vi "Send DB Data.vi"(0 "error in":errorcluster) -> ()   [LabVIEW 2012]
uses:
  Systems/Cannon/Cannon Global Data.vi
  Systems/Conveyer Belt/Conveyer Belt Global Data.vi
  Systems/Drive/Or David (Drive Global Data).vi
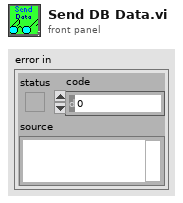
[diagram p1: front panel]
types:
  T1 = cluster{"Throttle":dbl, "RPM":dbl, "Motor VBus":dbl}
  T2 = cluster{"Horizontal Belt":dbl, "Vertical Belt":dbl, "MS":bool}
  T3 = typedef "WPI_SolenoidValue.ctl" = enum16{"Off", "On", "Forward", "Reverse"}
  T4 = cluster{"Shifter?":bool, "Axisses":dbl[], "Shifter Value":T3}
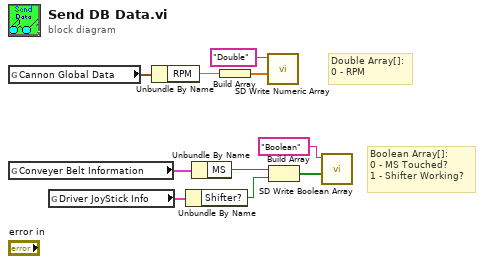
[diagram p0: block diagram]
diagram:
  # "Boolean Array[]:\n0 - MS Touched?\n1 - Shifter Working?"
  # "Double Array[]:\n0 - RPM"
  n1 = global read "Cannon Global Data.vi" "Cannon Global Data"() -> (w8:T1)
  n2 = global read "Conveyer Belt Global Data.vi" "Conveyer Belt Information"() -> (w5:T2)
  n3 = global read "Or David (Drive Global Data).vi" "Driver JoyStick Info"() -> (w4:T4)
  n4 = Unbundle By Name(w8) -> ("RPM"=w7:dbl)
  n5 = Unbundle By Name(w4) -> ("Shifter?"=w2:bool)
  n6 = Unbundle By Name(w5) -> ("MS"=w3:bool)
  n7 = Build Array(w7) -> (w6:dbl[])
  n8 = call <vilib>:"SD Write Numeric Array.vi"("Numeric Array"=w6, "Name"="Double") -> ()  [unwired: 8 in, 2 out]
  n9 = Build Array(w3, w2) -> (w1:bool[])
  n10 = call <vilib>:"SD Write Boolean Array.vi"("Boolean Array"=w1, "Name"="Boolean") -> ()  [unwired: 8 in, 2 out]
